vi "Extract Multiple Tone Information N Chan - N Specs (CDB).vi"(0 "time signals in":waveform(cdb)[](array[waveform]), 5 "export mode":T3(array[ring]), 7 "threshold":dbl[](array[numeric]) format="%#_6p", 9 "max num tones":i32[](array[numeric]), 11 "error in (no error)":errorcluster, 12 "output sorting":i32(ring) items=["increasing frequency", "decreasing amplitude"]) -> (3 "exported signals":T1(array[cluster]) {"exported spectrum (dB)"."dB Spectrum (Hann)" format="%.2p"; "exported spectrum (dB)"."df" format="%.2p"; "exported spectrum (dB)"."f0" format="%.2p"}, 4 "multiple tone information":T2(array[cluster]) {"multiple tone information"."detected phase (deg)" format="%_6g"; "multiple tone information"."detected amplitude" format="%_6p"; "multiple tone information"."detected frequency" format="%_6p"}, 15 "error out":errorcluster)   [LabVIEW 2020, in "NI_MAPro.lvlib"]
doc: "Returns the frequency, amplitude, and phase for each signal tone whose amplitude exceeds a specified <B>threshold</B>. Wire data to the <B>time signal in</B> input to determine the polymorphic instance to use or manually select the instance."
uses:
  NI_MAPro.lvlib
  NI_MABase.lvlib
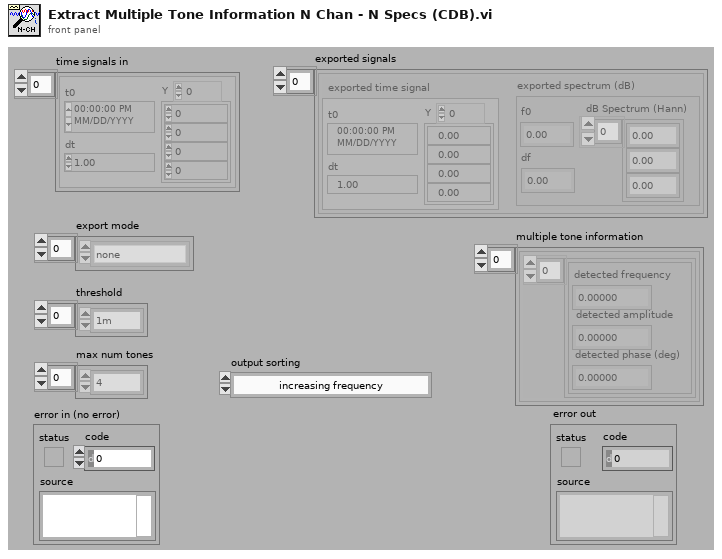
[diagram p1: front panel]
types:
  T1 = cluster{"exported time signal":waveform(cdb), "exported spectrum (dB)":cluster{"f0":dbl, "df":dbl, "dB Spectrum (Hann)":dbl[]}}[]
  T2 = cluster{"multiple tone information":cluster{"detected frequency":dbl, "detected amplitude":dbl, "detected phase (deg)":dbl}[]}[]
  T3 = enum32{"none", "input signal", "detected signal", "residual signal"}[]
  T4 = cluster{"exported time signal":waveform(cdb), "exported spectrum (dB)":cluster{"f0":dbl, "df":dbl, "dB Spectrum (Hann)":dbl[]}}
  T5 = cluster{"detected frequency":dbl, "detected amplitude":dbl, "detected phase (deg)":dbl}[]
  T6 = cluster{"multiple tone information":cluster{"detected frequency":dbl, "detected amplitude":dbl, "detected phase (deg)":dbl}[]}
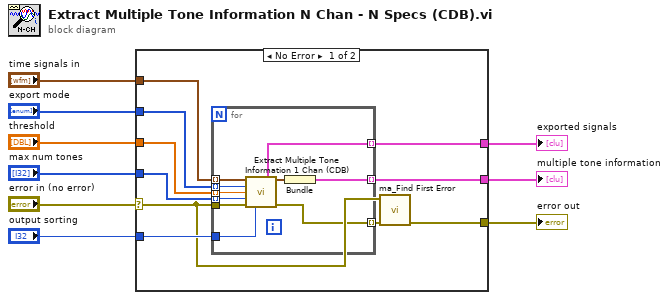
[diagram p0: block diagram]
diagram:
  n1 = case shown="No Error" "error in (no error)" {
    selector: "error in (no error)" -> [w12 w30]
    tunnel: "output sorting" -> [w19 _]
    tunnel: "time signals in" -> [w18 _]
    tunnel: [w16 w30] -> w7
    tunnel: "export mode" -> [w15 _]
    tunnel: "threshold" -> [w14 _]
    tunnel: "max num tones" -> [w13 _]
    tunnel: [w11 _] -> w2
    tunnel: [w10 _] -> w1
    frame No Error {
      n2 = for {
        tunnel: w12 -> [w29]
        tunnel: w13 -> [w28] mode=indexing
        tunnel: w14 -> [w27] mode=indexing
        tunnel: w15 -> [w26] mode=indexing
        tunnel: w19 -> [w25]
        tunnel: w18 -> [w24] mode=indexing
        tunnel: [w23] -> w11 mode=indexing
        tunnel: [w21] -> w10 mode=indexing
        tunnel: [w20] -> w17 mode=indexing
        n3 = call "Extract Multiple Tone Information 1 Chan (CDB).vi"("time signal in"=w24, "export mode"=w26, "threshold"=w27, "max num tones"=w28, "error in (no error)"=w29, "output sorting"=w25) -> ("exported signals"=w23:T4, "multiple tone information"=w22:T5, "error out"=w20:errorcluster)  [unwired: 7 out]
        n4 = Bundle("multiple tone information"=w22) -> (w21:T6)  [unwired: 1 in]
      }
      n5 = call "ma_Find First Error.vi"("error array in"=w17, "error in 1 (no error)"=w12) -> ("error out"=w16:errorcluster)  [unwired: 2 in, 3 out]
    }
    frame Error {
    }
  }
  "error out" <- w7
  "exported signals" <- w2
  "multiple tone information" <- w1
